vi "API Tester.vi"() -> ()   [LabVIEW 2020]
uses:
  Controls/test_property Type.ctl
  Controls/FlexLogger File Name and Path.ctl
  Controls/FlexLogger Session State Enum.ctl
  Controls/Flexlogger Data Rate Level Enum.ctl
  FlexLogger_gRPC.lvclass
panel:
  in  "channel_name 2":string caption="channel_name"
  in  "Set Data Rate":bool
  in  "Data Rate Level":T1
  in  "channel_name":string
  in  "Get Data Rate":bool
  out "Data Rate Level":T1
  out "document_identifier":T2
  in  "Get Log Spec. Doc.":bool
  in  "Get Curr Project":bool
  out "SetLogFile":bool caption="Set LogFileNameAndPath"
  out "ReadLogFile":bool caption="Read LogFileNameAndPath"
  out "AddNote":bool
  in  "Get Log File Path":bool
  in  "Get Session Time":bool
  in  "Get Session State":bool
  in  "Connect":bool
  in  "Read Property":bool
  in  "Write Property":bool
  in  "Add Note":bool
  in  "Start Test":bool
  in  "Stop Test":bool
  in  "Read All Properties":bool
  in  "Note":string
  in  "Close Connection":bool
  in  "Property Name":string="Operator"
  out "Property Read":T3
  out "Test_Properties Array":T3[](array[typedef])
  in  "PropertyName":string="DUT"
  in  "PropertyValue":string="EV Battery"
  in  "Remove Property":bool
  out "LogFileNamePath Read":T4
  in  "LogFileNamePath Set":T4={"File Path"="LogFile_{Year}-{Month}-{Day}-{Hour}-{Minute}-{Second}.tdms", "File Name"="C:\\Users\\Documents\\FlexLogger\\dataTest", "Resolved File Path"="LogFile_2021-11-07-21-36-12.tdms", "Resolved File Name"="C:\\Users\\Documents\\FlexLogger\\data"}
  in  "Set Log File Path":bool
  in  "Open Project":bool
  in  "Close Project":bool
  out "Session\nState":T5=enum."Idle"
  out "Elapsed\nTime":i32
  out "Connectted":bool caption="Connect"
  out "OpenProject":bool
  out "StartTest":bool
  out "StopTest":bool
  out "CloseProject":bool
  out "Disconnect":bool
  out "Response Data":T6
  in  "FlexLoggerProjPath":path
  # "FlexLogger GRPC Control"
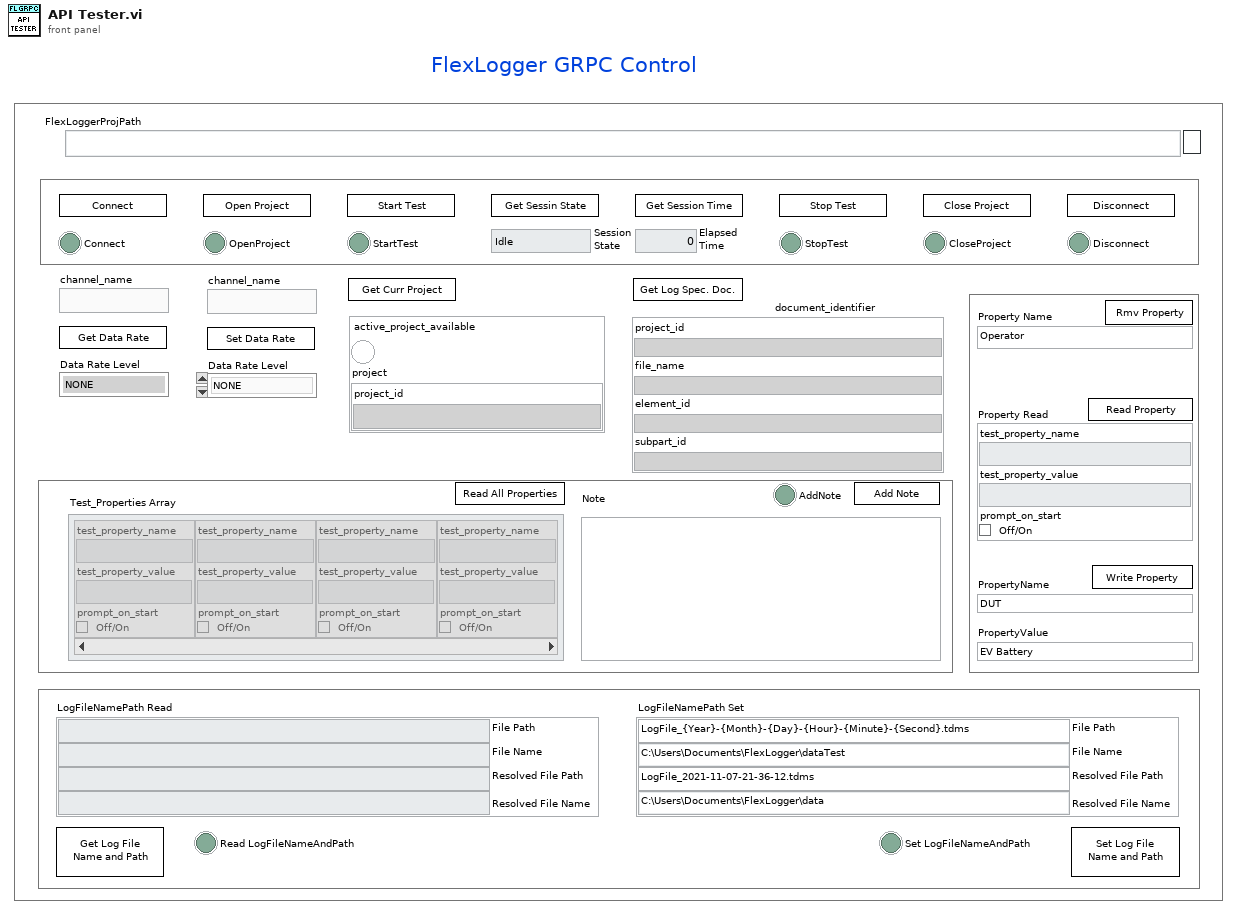
[diagram p1: front panel]
types:
  T1 = typedef "FlexLogger_gRPC.lvlib/FlexLogger_gRPC.lvclass/Flexlogger Data Rate Level Enum.ctl" = enum16{"NONE", "SLOW", "MEDIUM", "FAST", "COUNTER", "DIGITAL", "ON DEMAND"}
  T2 = cluster{"project_id":string, "file_name":string, "element_id":string, "subpart_id":string}
  T3 = typedef "FlexLogger_gRPC.lvlib/FlexLogger_gRPC.lvclass/test_property Type.ctl" = cluster{"test_property_name":string, "test_property_value":string, "prompt_on_start":bool}
  T4 = typedef "FlexLogger_gRPC.lvlib/FlexLogger_gRPC.lvclass/FlexLogger File Name and Path.ctl" = cluster{"File Path":string, "File Name":string, "Resolved File Path":string, "Resolved File Name":string}
  T5 = typedef "FlexLogger_gRPC.lvlib/FlexLogger_gRPC.lvclass/FlexLogger Session State Enum.ctl" = enum16{"Unknown", "Idle", "Running", "Invalid Configuration", "No Valid Logged Channels", "Paused"}
  T6 = cluster{"active_project_available":bool, "project":cluster{"project_id":string}}
  T7 = typedef "FlexLogger_client.lvlib/flexlogger_GetActiveProjectResponse.ctl" = cluster{"active_project_available":bool, "project":T8}
  T8 = typedef "FlexLogger_client.lvlib/flexlogger_ProjectIdentifier.ctl" = cluster{"project_id":string}
  T9 = typedef "FlexLogger_client.lvlib/flexlogger_ElementIdentifier.ctl" = cluster{"project_id":string, "file_name":string, "element_id":string, "subpart_id":string}
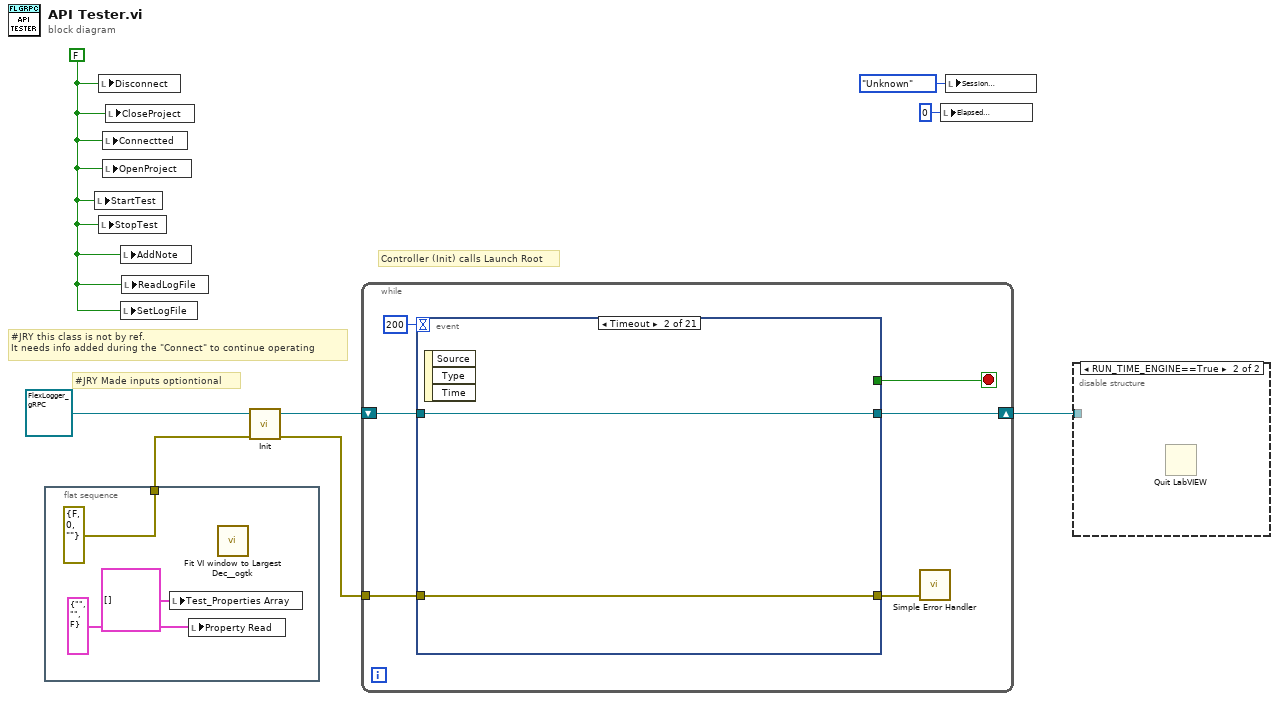
[diagram p0: block diagram]
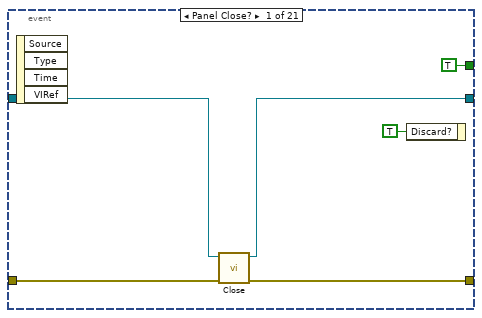
[diagram p3: hidden frame]
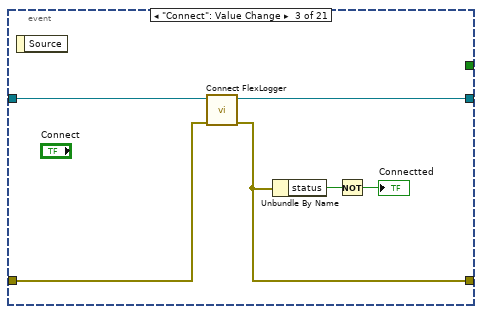
[diagram p4: hidden frame]
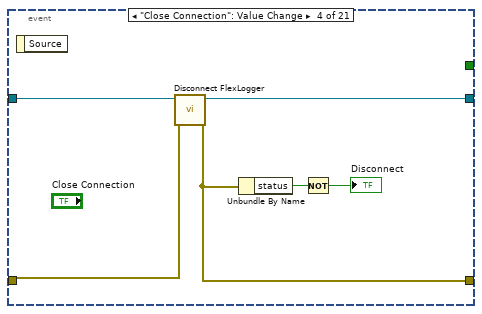
[diagram p5: hidden frame]
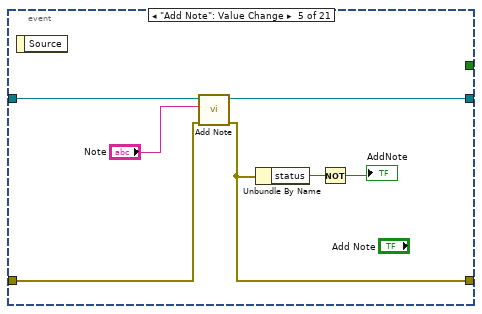
[diagram p6: hidden frame]
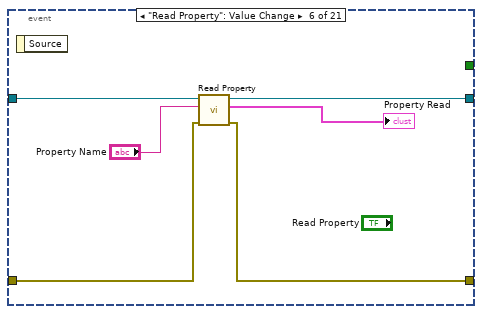
[diagram p7: hidden frame]
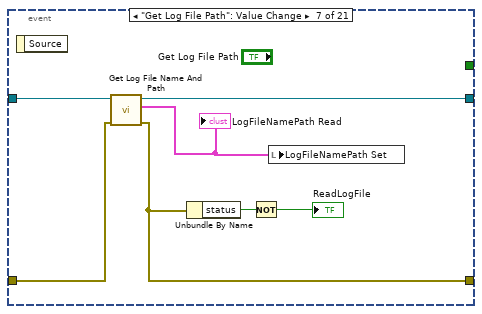
[diagram p8: hidden frame]
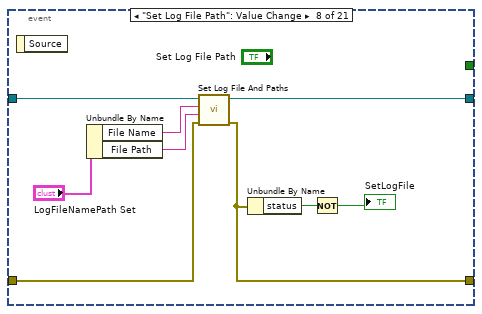
[diagram p9: hidden frame]
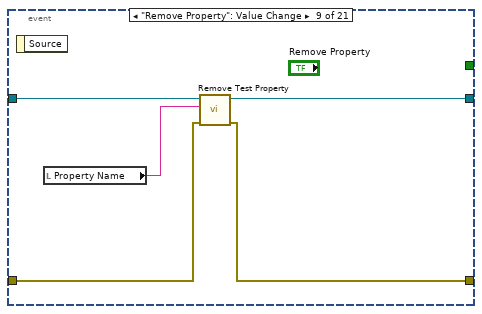
[diagram p10: hidden frame]
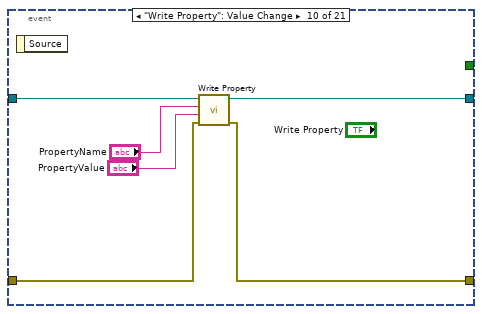
[diagram p11: hidden frame]
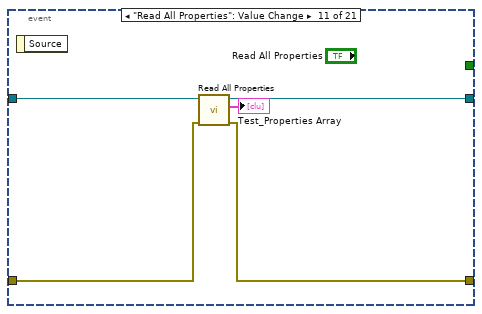
[diagram p12: hidden frame]
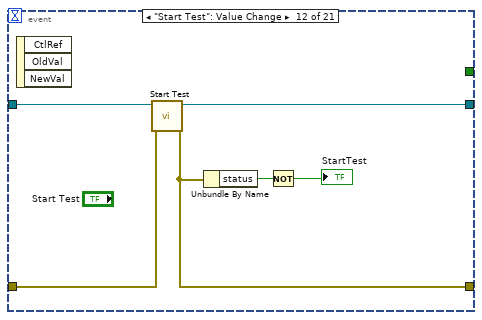
[diagram p13: hidden frame]
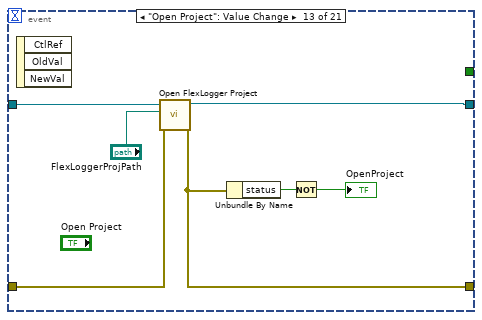
[diagram p14: hidden frame]
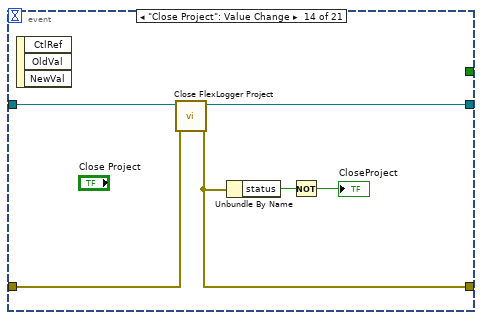
[diagram p15: hidden frame]
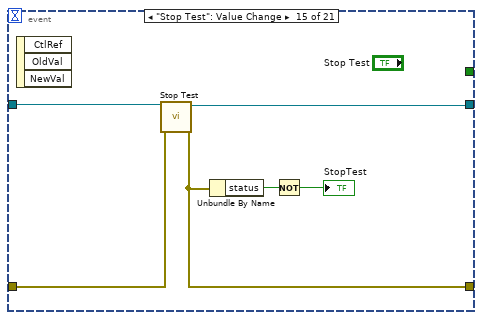
[diagram p16: hidden frame]
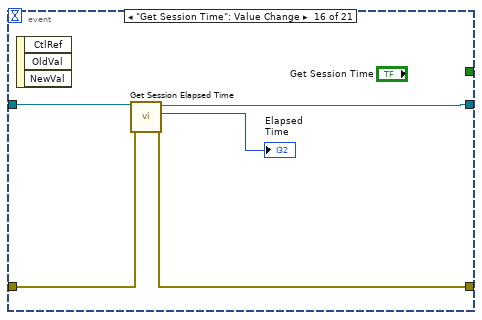
[diagram p17: hidden frame]
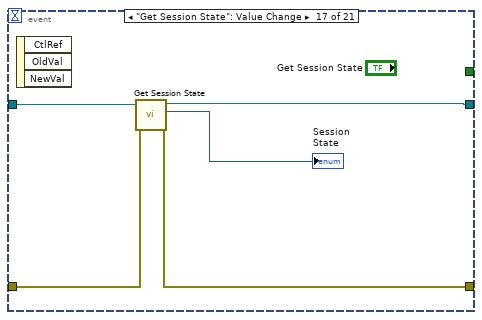
[diagram p18: hidden frame]
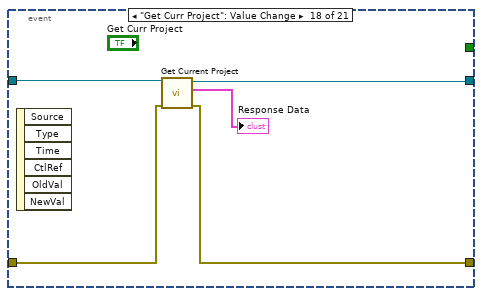
[diagram p19: hidden frame]
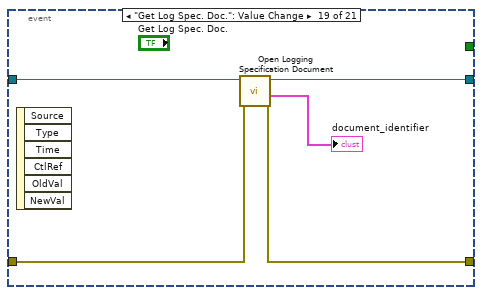
[diagram p20: hidden frame]
diagram:
  w5 = FALSE ("Stop")
  # "#JRY this class is not by ref.\nIt needs info added during the \"Connect\" to continue operating"
  # "#JRY Made inputs optiontional"
  # "Controller (Init) calls Launch Root"
  n1 = flat-sequence {
    tunnel: [errorcluster {"status"=FALSE, "code"=0, "source"=""} ("error constant")] -> w2
    frame #0 {
      n2 = local write "Test_Properties Array"(T3[] [] ("Test_Properties Array")) -> ()
      n3 = local write "Property Read"(T3 {"test_property_name"="", "test_property_value"="", "prompt_on_start"=FALSE} ("Property Read")) -> ()
      n4 = call <userlib>:"Fit VI window to Largest Dec__ogtk.vi"() -> ()  [unwired: 6 in, 2 out]
    }
  }
  n5 = local write "StartTest"(w5) -> ()
  n6 = local write "Disconnect"(w5) -> ()
  n7 = local write "StopTest"(w5) -> ()
  n8 = local write "Connectted"(w5) -> ()
  n9 = local write "OpenProject"(w5) -> ()
  n10 = local write "CloseProject"(w5) -> ()
  n11 = local write "AddNote"(w5) -> ()
  n12 = local write "SetLogFile"(w5) -> ()
  n13 = local write "ReadLogFile"(w5) -> ()
  n14 = call-dynamic "Init.vi"("error in (no error)"=w2, "FlexLogger_gRPCAPI in"=refnum<class "FlexLogger_gRPC.lvclass"> refnum ("FlexLogger_gRPC.lvlib:FlexLogger_gRPC.lvclass")) -> ("error out"=w7:errorcluster, "FlexLogger_gRPCAPI out"=w8:refnum<class "FlexLogger_gRPC.lvclass">)  [unwired: 8 in]
  n15 = while {
    shift-right: [w13] -> w6
    shift-left: w8 -> [w15]
    tunnel: w7 -> [w16]
    stop <- w17 stop-if-true
    n16 = event shown="[1] Timeout" {
      selector: _ -> [_ _ _ _ _ _ _ _ _ _ _ _ _ _ _ _ _ _ _ _ _]
      dyn-events: _ -> [_ _ _ _ _ _ _ _ _ _ _ _ _ _ _ _ _ _ _ _ _]
      timeout: 200 -> [_ _ _ _ _ _ _ _ _ _ _ _ _ _ _ _ _ _ _ _ _]
      tunnel: [TRUE ("Stop 2") _ _ _ _ _ _ _ _ _ _ _ _ _ _ _ _ _ _ _ _] -> w17
      tunnel: w16 -> [w23 w24 w29 w35 w43 w49 w56 w65 w70 w76 w81 w87 w94 w100 w106 w111 w116 w121 w126 w131 w137]
      tunnel: w15 -> [w22 w25 w31 w37 w44 w50 w57 w66 w71 w77 w82 w88 w95 w101 w107 w112 w117 w122 w127 w133 w139]
      tunnel: [w20 w24 w27 w33 w39 w48 w52 w59 w69 w75 w80 w84 w92 w97 w103 w110 w115 w120 w124 w130 w136] -> w12
      tunnel: [w21 w25 w30 w36 w41 w46 w54 w61 w67 w72 w78 w86 w93 w99 w105 w108 w113 w119 w125 w132 w138] -> w13
      event Panel Close? {
        n17 = event-data() -> ()  [unwired: 1 in, 4 out]
        n18 = call-dynamic "Close.vi"("error in (no error)"=w23, "FlexLogger_gRPC in"=w22) -> ("error out"=w20:errorcluster, "FlexLogger_gRPC out"=w21:refnum<class "FlexLogger_gRPC.lvclass">)  [unwired: 8 in]
        n19 = event-data("Discard?"=TRUE) -> ()  [unwired: 1 in, 1 out]
      }
      event Timeout {
        n20 = event-data() -> ()  [unwired: 1 in, 3 out]
      }
      event "Connect": Value Change {
        n21 = event-data() -> ()  [unwired: 1 in, 1 out]
        n22 = call-dynamic "Connect FlexLogger.vi"("error in (no error)"=w29, "FlexLogger_gRPCAPI in"=w31) -> ("error out"=w27:errorcluster, "FlexLogger_gRPCAPI out"=w30:refnum<class "FlexLogger_gRPC.lvclass">)  [unwired: 8 in]
        n23 = Unbundle By Name(w27) -> ("status"=w28:bool)
        n24 = Not(x=w28) -> (.not. x?=→"Connectted":bool)
      }
      event "Close Connection": Value Change {
        n25 = event-data() -> ()  [unwired: 1 in, 1 out]
        n26 = call-dynamic "Disconnect FlexLogger.vi"("error in (no error)"=w35, "FlexLogger_gRPCAPI in"=w37) -> ("error out"=w33:errorcluster, "FlexLogger_gRPCAPI out"=w36:refnum<class "FlexLogger_gRPC.lvclass">)  [unwired: 8 in]
        n27 = Unbundle By Name(w33) -> ("status"=w34:bool)
        n28 = Not(x=w34) -> (.not. x?=→"Disconnect":bool)
      }
      event "Add Note": Value Change {
        n29 = event-data() -> ()  [unwired: 1 in, 1 out]
        n30 = call-dynamic "Add Note.vi"("error in (no error)"=w43, "Note"="Note", "FlexLogger_gRPCAPI in"=w44) -> ("error out"=w39:errorcluster, "FlexLogger_gRPCAPI out"=w41:refnum<class "FlexLogger_gRPC.lvclass">)  [unwired: 7 in]
        n31 = Unbundle By Name(w39) -> ("status"=w40:bool)
        n32 = Not(x=w40) -> (.not. x?=→"AddNote":bool)
      }
      event "Read Property": Value Change {
        n33 = event-data() -> ()  [unwired: 1 in, 1 out]
        n34 = call-dynamic "Read Property.vi"("error in (no error)"=w49, "property name"="Property Name", "FlexLogger_gRPCAPI in"=w50) -> ("error out"=w48:errorcluster, "Test_Properties Array"=→"Property Read":T3, "FlexLogger_gRPCAPI out"=w46:refnum<class "FlexLogger_gRPC.lvclass">)  [unwired: 6 in]
      }
      event "Get Log File Path": Value Change {
        n35 = event-data() -> ()  [unwired: 1 in, 1 out]
        n36 = call-dynamic "Get Log File Name And Path.vi"("error in (no error)"=w56, "FlexLogger_gRPCAPI in"=w57) -> ("error out"=w52:errorcluster, "LogFileNamePath"=w55:T4, "FlexLogger_gRPCAPI out"=w54:refnum<class "FlexLogger_gRPC.lvclass">)  [unwired: 7 in]
        "LogFileNamePath Read" <- w55
        n37 = Unbundle By Name(w52) -> ("status"=w53:bool)
        n38 = Not(x=w53) -> (.not. x?=→"ReadLogFile":bool)
        n39 = local write "LogFileNamePath Set"(w55) -> ()
      }
      event "Set Log File Path": Value Change {
        n40 = event-data() -> ()  [unwired: 1 in, 1 out]
        n41 = Unbundle By Name("LogFileNamePath Set") -> ("File Name"=w63:string, "File Path"=w62:string)
        n42 = call-dynamic "Set Log File And Paths.vi"("error in (no error)"=w65, "File Path"=w62, "File Name"=w63, "FlexLogger_gRPCAPI in"=w66) -> ("error out"=w59:errorcluster, "FlexLogger_gRPCAPI out"=w61:refnum<class "FlexLogger_gRPC.lvclass">)  [unwired: 6 in]
        n43 = Unbundle By Name(w59) -> ("status"=w60:bool)
        n44 = Not(x=w60) -> (.not. x?=→"SetLogFile":bool)
      }
      event "Remove Property": Value Change {
        n45 = event-data() -> ()  [unwired: 1 in, 1 out]
        n46 = local read "Property Name"() -> (w68:string)
        n47 = call-dynamic "Remove Test Property.vi"("error in (no error)"=w70, "testPropertyName"=w68, "FlexLogger_gRPCAPI in"=w71) -> ("error out"=w69:errorcluster, "FlexLogger_gRPCAPI out"=w67:refnum<class "FlexLogger_gRPC.lvclass">)  [unwired: 7 in]
      }
      event "Write Property": Value Change {
        n48 = event-data() -> ()  [unwired: 1 in, 1 out]
        n49 = call-dynamic "Write Property.vi"("error in (no error)"=w76, "Property Value"="PropertyValue", "Property Name"="PropertyName", "FlexLogger_gRPCAPI in"=w77) -> ("error out"=w75:errorcluster, "FlexLogger_gRPCAPI out"=w72:refnum<class "FlexLogger_gRPC.lvclass">)  [unwired: 6 in]
      }
      event "Read All Properties": Value Change {
        n50 = event-data() -> ()  [unwired: 1 in, 1 out]
        n51 = call-dynamic "Read All Properties.vi"("error in (no error)"=w81, "FlexLogger_gRPCAPI in"=w82) -> ("error out"=w80:errorcluster, "Test_Properties Array"=→"Test_Properties Array":T3[], "FlexLogger_gRPCAPI out"=w78:refnum<class "FlexLogger_gRPC.lvclass">)  [unwired: 7 in]
      }
      event "Start Test": Value Change {
        n52 = event-data() -> ()  [unwired: 1 in, 3 out]
        n53 = call-dynamic "Start Test.vi"("error in (no error)"=w87, "FlexLogger_gRPCAPI in"=w88) -> ("error out"=w84:errorcluster, "FlexLogger_gRPCAPI out"=w86:refnum<class "FlexLogger_gRPC.lvclass">)  [unwired: 7 in, 1 out]
        n54 = Unbundle By Name(w84) -> ("status"=w85:bool)
        n55 = Not(x=w85) -> (.not. x?=→"StartTest":bool)
      }
      event "Open Project": Value Change {
        n56 = event-data() -> ()  [unwired: 1 in, 3 out]
        n57 = call-dynamic "Open FlexLogger Project.vi"("error in (no error)"=w94, "FlexLoggerProjPath in"="FlexLoggerProjPath", "FlexLogger_gRPCAPI in"=w95) -> ("error out"=w92:errorcluster, "FlexLogger_gRPCAPI out"=w93:refnum<class "FlexLogger_gRPC.lvclass">)  [unwired: 6 in, 1 out]
        n58 = Unbundle By Name(w92) -> ("status"=w91:bool)
        n59 = Not(x=w91) -> (.not. x?=→"OpenProject":bool)
      }
      event "Close Project": Value Change {
        n60 = event-data() -> ()  [unwired: 1 in, 3 out]
        n61 = call-dynamic "Close FlexLogger Project.vi"("error in (no error)"=w100, "FlexLogger_gRPCAPI in"=w101) -> ("error out"=w97:errorcluster, "FlexLogger_gRPCAPI out"=w99:refnum<class "FlexLogger_gRPC.lvclass">)  [unwired: 7 in, 1 out]
        n62 = Unbundle By Name(w97) -> ("status"=w98:bool)
        n63 = Not(x=w98) -> (.not. x?=→"CloseProject":bool)
      }
      event "Stop Test": Value Change {
        n64 = event-data() -> ()  [unwired: 1 in, 3 out]
        n65 = call-dynamic "Stop Test.vi"("error in (no error)"=w106, "FlexLogger_gRPCAPI in"=w107) -> ("error out"=w103:errorcluster, "FlexLogger_gRPCAPI out"=w105:refnum<class "FlexLogger_gRPC.lvclass">)  [unwired: 8 in]
        n66 = Unbundle By Name(w103) -> ("status"=w104:bool)
        n67 = Not(x=w104) -> (.not. x?=→"StopTest":bool)
      }
      event "Get Session Time": Value Change {
        n68 = event-data() -> ()  [unwired: 1 in, 3 out]
        n69 = call-dynamic "Get Session Elapsed Time.vi"("error in (no error)"=w111, "FlexLogger_gRPCAPI in"=w112) -> ("error out"=w110:errorcluster, "Elapsed Time"=→"Elapsed\nTime":i32, "FlexLogger_gRPCAPI out"=w108:refnum<class "FlexLogger_gRPC.lvclass">)  [unwired: 7 in]
      }
      event "Get Session State": Value Change {
        n70 = event-data() -> ()  [unwired: 1 in, 3 out]
        n71 = call-dynamic "Get Session State.vi"("error in (no error)"=w116, "FlexLogger_gRPCAPI in"=w117) -> ("error out"=w115:errorcluster, "Session State"=→"Session\nState":T5, "FlexLogger_gRPCAPI out"=w113:refnum<class "FlexLogger_gRPC.lvclass">)  [unwired: 7 in]
      }
      event "Get Curr Project": Value Change {
        n72 = event-data() -> ()  [unwired: 1 in, 6 out]
        n73 = call-dynamic "Get Current Project.vi"("error in (no error)"=w121, "FlexLogger_gRPC in"=w122) -> ("error out"=w120:errorcluster, "Response Data"=→"Response Data":T7, "FlexLogger_gRPC out"=w119:refnum<class "FlexLogger_gRPC.lvclass">)  [unwired: 7 in]
      }
      event "Get Log Spec. Doc.": Value Change {
        n74 = event-data() -> ()  [unwired: 1 in, 6 out]
        n75 = call-dynamic "Open Logging Specification Document.vi"("error in (no error)"=w126, "FlexLogger_gRPC in"=w127) -> ("error out"=w124:errorcluster, "document_identifier"=→"document_identifier":T9, "FlexLogger_gRPC out"=w125:refnum<class "FlexLogger_gRPC.lvclass">)  [unwired: 7 in]
      }
      event "Get Data Rate": Value Change {
        n76 = event-data() -> ()  [unwired: 1 in, 6 out]
        n77 = call-dynamic "Get DataRateLevel.vi"("error in (no error)"=w131, "channel_name"="channel_name", "FlexLogger_gRPC in"=w133) -> ("error out"=w130:errorcluster, "Data Rate Level"=→"Data Rate Level":T1, "FlexLogger_gRPC out"=w132:refnum<class "FlexLogger_gRPC.lvclass">)  [unwired: 6 in]
      }
      event "Set Data Rate": Value Change {
        n78 = event-data() -> ()  [unwired: 1 in, 6 out]
        n79 = call-dynamic "Set DataRateLevel.vi"("error in (no error)"=w137, "channel_name"="channel_name 2", "Data Rate Level"="Data Rate Level", "FlexLogger_gRPC in"=w139) -> ("error out"=w136:errorcluster, "FlexLogger_gRPC out"=w138:refnum<class "FlexLogger_gRPC.lvclass">)  [unwired: 6 in]
      }
    }
    n80 = call <vilib>:"Simple Error Handler.vi"("error in (no error)"=w12) -> ()  [unwired: 4 in, 5 out]
  }
  n81 = local write "Elapsed\nTime"(0 ("Elapsed\nTime")) -> ()
  n82 = local write "Session\nState"(FlexLogger_Session_State_Enum."Unknown" ("Session\nState")) -> ()
  n83 = disable-structure shown="RUN_TIME_ENGINE==True" {
    disable-tunnel: w6 -> [_ _]
    frame condition #0 (active) {
    }
    frame condition #1 {
      n84 = Quit LabVIEW() -> ()  [unwired: 1 in]
    }
  }
